vi "pathplan.vi"   [LabVIEW 2016]
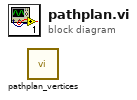
[diagram p0: block diagram]
diagram:
  n1 = call "pathplan_vertices.vi"() -> ()  [unwired: 9 in, 2 out]
